vi "Handle Last Ack Core.vi"(4 "error in (no error)":errorcluster, 6 "Last Ack":refnum<class "Last Ack.lvclass">, 7 "IMAQdx Actor in":refnum<class "IMAQdx Actor.lvclass">) -> (0 "error out":errorcluster, 3 "IMAQdx Actor out":refnum<class "IMAQdx Actor.lvclass">)   [LabVIEW 2014, in "IMAQdx Actor.lvlib" / "IMAQdx Actor.lvclass"]
doc: "(<B>Filename</B>: Actor Framework.lvlib:Actor.lvclass:Handle Last Ack Core.vi)\n\nDefines how the caller actor responds to the Last Ack message from a nested actor. The Last Ack message is the final message a nested actor sends to its caller before it shuts down. The message contains information about the final state of the nested actor.\n\nBy default, this method does nothing except return any error the nested actor sent. A descendant class may override this method to define behavior."
uses:
  IMAQdx Actor.lvclass
  <vilib>/ActorFramework/LastAck/Last Ack.lvclass
  <vilib>/ActorFramework/Message Enqueuer/Message Enqueuer.lvclass
  Camera Settings Dialog/Camera Settings Dialog/Camera Settings Dialog.lvclass
  <vilib>/ActorFramework/LastAck/Last Ack.lvclass/Last Ack.ctl
  IMAQdx Actor.lvclass/IMAQdx Actor.ctl
  Camera Actor/Camera Actor/Camera Actor.lvclass
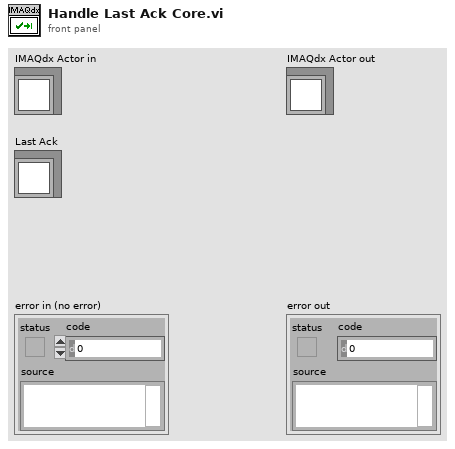
[diagram p1: front panel]
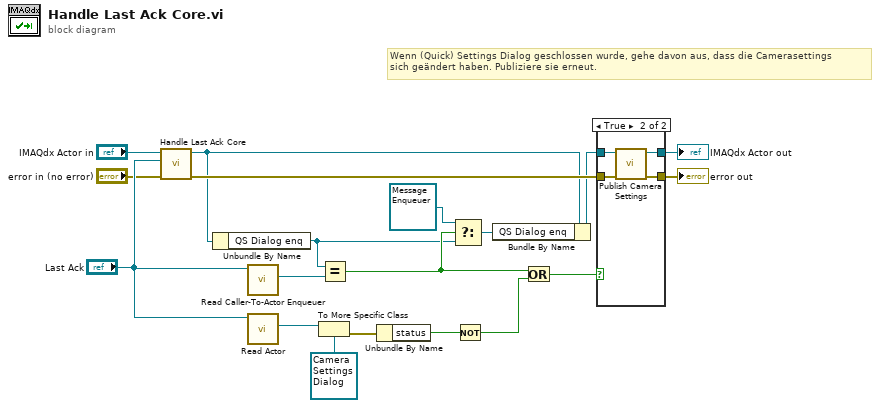
[diagram p0: block diagram]
diagram:
  # "Wenn (Quick) Settings Dialog geschlossen wurde, gehe davon aus, dass die Camerasettings\nsich geändert haben. Publiziere sie erneut."
  n1 = call-parent "Handle Last Ack Core.vi"("error in (no error)"="error in (no error)", "Last Ack"="Last Ack", "Actor in"="IMAQdx Actor in") -> ("error out"=w17:errorcluster, "Actor out"=w14:refnum<class "IMAQdx Actor.lvclass">)  [unwired: 3 in]
  n2 = Unbundle By Name(w14) -> ("QS Dialog enq"=w11:refnum<class "Message Enqueuer.lvclass">)
  n3 = call <vilib>:"Read Caller-To-Actor Enqueuer.vi"("Last Ack"="Last Ack") -> ("Caller-to-Actor Enqueuer"=w13:refnum<class "Message Enqueuer.lvclass">)  [unwired: 10 in]
  n4 = call <vilib>:"Read Actor.vi"("Last Ack"="Last Ack") -> ("Actor"=w6:refnum<class "Actor.lvclass">)  [unwired: 10 in]
  n5 = To More Specific Class(target class=refnum<class "Camera Settings Dialog.lvclass"> refnum ("Camera Settings Dialog.lvlib:Camera Settings Dialog.lvclass"), reference=w6) -> (error out=w4:errorcluster)  [unwired: 1 in, 1 out]
  n6 = Equal?(x=w11, y=w13) -> (x = y?=w18:bool)
  n7 = Unbundle By Name(w4) -> ("status"=w2:bool)
  n8 = Select(t=refnum<class "Message Enqueuer.lvclass"> refnum, s=w18, f=w11) -> (s? t:f=w12:refnum<class "Message Enqueuer.lvclass">)
  n9 = Not(x=w2) -> (.not. x?=w1:bool)
  n10 = Bundle By Name(cluster=w14, "QS Dialog enq"=w12) -> (w8:refnum<class "IMAQdx Actor.lvclass">)
  n11 = Or(x=w18, y=w1) -> (x .or. y?=w3:bool)
  n12 = case shown="True" w3 {
    tunnel: w17 -> [w20 w25]
    tunnel: [w20 w24] -> w9
    tunnel: w8 -> [w21 w23]
    tunnel: [w21 w22] -> w7
    frame False {
    }
    frame True {
      n13 = call-dynamic "Publish Camera Settings.vi"("error in (no error)"=w25, "IMAQdx Actor in"=w23) -> ("error out"=w24:errorcluster, "IMAQdx Actor out"=w22:refnum<class "IMAQdx Actor.lvclass">)  [unwired: 8 in]
    }
  }
  "IMAQdx Actor out" <- w7
  "error out" <- w9
